vi "NI VeriStand - Get Custom Device Channel Value Table.vi"(8 "error in (no error)":errorcluster, 11 "Channel Ref in":T1 format="%.0x") -> (0 "error out":errorcluster, 1 "Values":dbl[](array[numeric]), 2 "Names":string[](array[string]), 3 "Channel Ref out":T1=18446744073709551615 format="%.0x")   [LabVIEW 2026, in "Custom Devices Storage.lvlib"]
uses:
  Custom Devices Storage.lvlib
  <vilib>/NI VeriStand/Custom Device API/Custom Device Item Ref.ctl
  C:/Users/Administrator/Desktop/Jatin/All DNC DLLs/NationalInstruments.VeriStand.SystemDefinitionAPI.dll
  Jatin/All DNC DLLs/NationalInstruments.VeriStand.SystemDefinitionAPI.dll
  C:/Users/Administrator/Desktop/Jatin/All DNC DLLs/NationalInstruments.VeriStand.SystemStorage.dll
  Jatin/All DNC DLLs/NationalInstruments.VeriStand.SystemStorage.dll
  <vilib>/NI VeriStand/Custom Device API/Custom Device API.lvlib
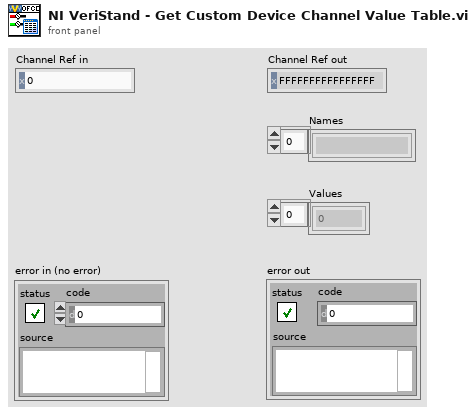
[diagram p1: front panel]
types:
  T1 = typedef "Custom Device API.lvlib/Custom Device Item Ref.ctl" = u64
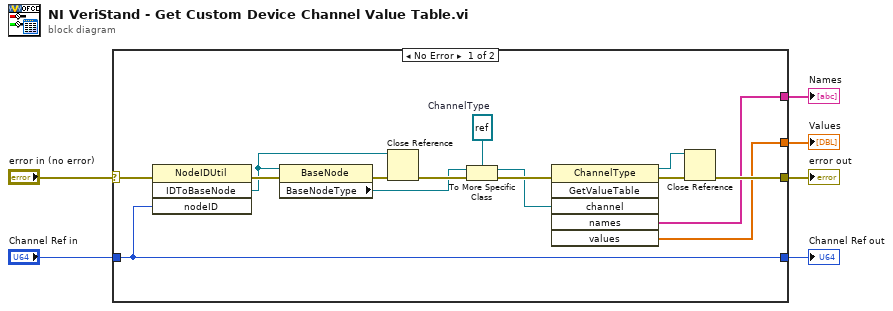
[diagram p0: block diagram]
diagram:
  n1 = case shown="No Error" "error in (no error)" {
    selector: "error in (no error)" -> [w18 w23]
    tunnel: [w17 w23] -> w5
    tunnel: "Channel Ref in" -> [w16 w22]
    tunnel: [w16 w22] -> w3
    tunnel: [w8 _] -> w2
    tunnel: [w7 _] -> w1
    frame No Error {
      w14 = refnum<k39> refnum  # ChannelType
      n2 = invoke class="NodeIDUtil" method="IDToBaseNode"(error in=w18, "nodeID"=w16) -> (error out=w21:errorcluster, "IDToBaseNode"=w19:refnum<k39>)  [unwired: 2 in, 2 out]
      n3 = property class="BaseNode"(reference=w19, error in=w21) -> (error out=w20:errorcluster, "BaseNodeType"=w11:refnum<k39>)  [unwired: 1 out]
      n4 = Close Reference(reference=w19, error in (no error)=w20) -> (error out=w12:errorcluster)
      n5 = To More Specific Class(target class=w14, reference=w11, error in=w12) -> (specific class reference=w13:refnum<k39>, error out=w15:errorcluster)
      n6 = invoke class="ChannelType" method="GetValueTable"(error in=w15, "channel"=w13) -> (reference out=w9:refnum<k39>, error out=w10:errorcluster, "names"=w8:string[], "values"=w7:dbl[])  [unwired: 4 in, 2 out]
      n7 = Close Reference(reference=w9, error in (no error)=w10) -> (error out=w17:errorcluster)
    }
    frame Error {
    }
  }
  "Channel Ref out" <- w3
  "error out" <- w5
  "Names" <- w2
  "Values" <- w1
